vi "Read CData.vi"(8 "error in (no error)":errorcluster, 11 "CData in":refnum<class "CData.lvclass">) -> (0 "error out":errorcluster, 2 "CData":T1, 3 "CData out":refnum<class "CData.lvclass">)   [LabVIEW 2014, in "CData.lvclass"]
uses:
  CData.lvclass
  Controls/CData Core Control.ctl
  CData.lvclass/CData.ctl
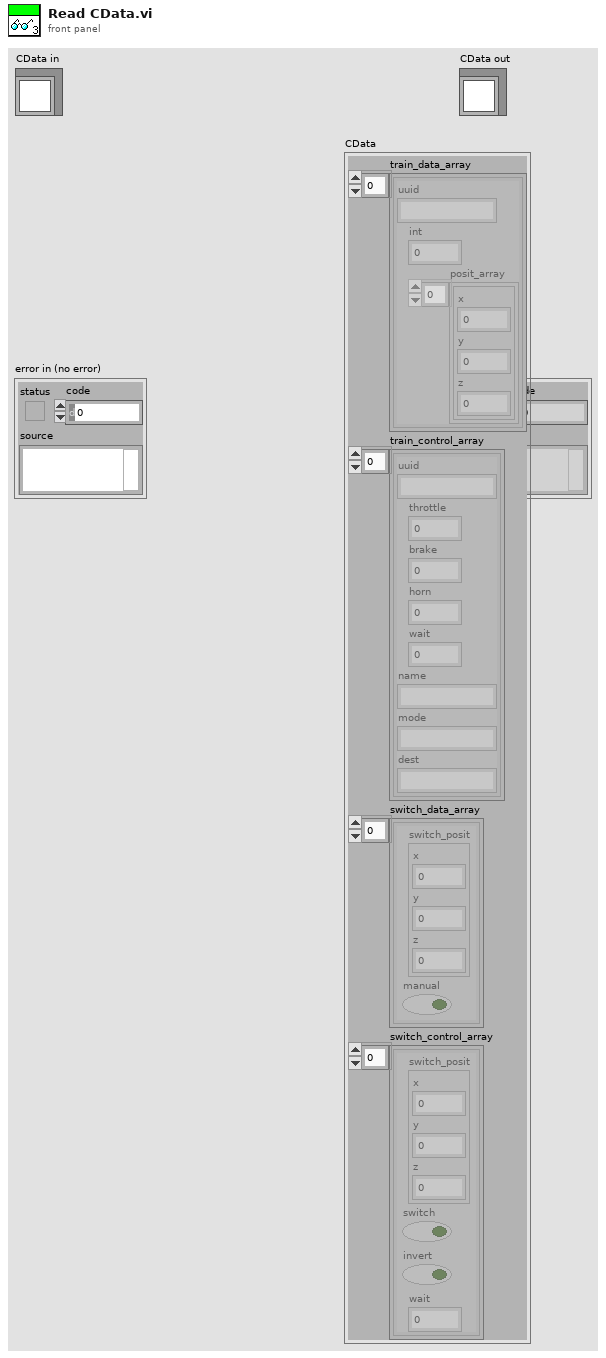
[diagram p1: front panel]
types:
  T1 = typedef "CData Core Control.ctl" = cluster{"train_data_array":cluster{"uuid":string, "int":i32, "posit_array":cluster{"x":dbl, "y":dbl, "z":dbl}[]}[], "train_control_array":cluster{"uuid":string, "throttle":dbl, "brake":dbl, "horn":dbl, "wait":dbl, "name":string, "mode":string, "dest":string}[], "switch_data_array":cluster{"switch_posit":cluster{"x":dbl, "y":dbl, "z":dbl}, "manual":bool}[], "switch_control_array":cluster{"switch_posit":cluster{"x":dbl, "y":dbl, "z":dbl}, "switch":bool, "invert":bool, "wait":dbl}[]}
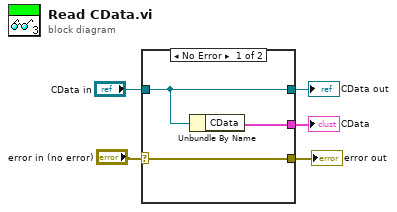
[diagram p0: block diagram]
diagram:
  n1 = case shown="No Error" "error in (no error)" {
    selector: "error in (no error)" -> [w8 w10]
    tunnel: [w8 w10] -> w4
    tunnel: [w7 w9] -> w2
    tunnel: "CData in" -> [w7 w9]
    tunnel: [w6 _] -> w1
    frame No Error {
      n2 = Unbundle By Name(w7) -> ("CData"=w6:T1)
    }
    frame Error {
    }
  }
  "error out" <- w4
  "CData out" <- w2
  "CData" <- w1
